vi "CRYPEAQ Makeing HarmonicTrack FlFcFu.vi"(10 "Harmonic Infor":T1={"Cycles"=[200.0, 190.0, 180.0, 170.0, 160.0, 150.0, 140.0, 132.0, 125.0, 118.0, 112.0, 106.0, 100.0, 95.0, 90.0, 85.0, 80.0, 75.0, 71.0, 67.0, 63.0, 60.0, 56.0, 53.0, 50.0, 48.0, 45.0, 43.0, 40.0, 38.0, 36.0, 34.0, 32.0, 30.0, 28.0, 27.0, 25.0, 24.0, 23.0, 22.0, 20.0, 19.0, 18.0, 17.0, 16.0, 15.0, 14.0, 14.0, 13.0, 12.0, 12.0, 11.0, 10.0, 10.0, 9.0, 9.0, 8.0, 8.0, 8.0, 7.0, 7.0, 6.0, 6.0, 6.0, 6.0, 6.0, 6.0, 6.0, 6.0, 6.0, 6.0, 6.0, 6.0, 6.0, 8.0, 8.0, 8.0, 8.0, 8.0, 8.0, 8.0, 8.0], "Frequency"=[20000.0, 19000.0, 18000.0, 17000.0, 16000.0, 15000.0, 14000.0, 13199.999809265137, 12500.0, 11800.000190734863, 11199.999809265137, 10600.000381469727, 10000.0, 9500.0, 9000.0, 8500.0, 8000.0, 7500.0, 7099.999904632568, 6699.999809265137, 6300.000190734863, 6000.0, 5599.999904632568, 5300.000190734863, 5000.0, 4750.0, 4500.0, 4250.0, 4000.0, 3750.0, 3549.999952316284, 3349.9999046325684, 3150.0000953674316, 3000.0, 2799.999952316284, 2650.0000953674316, 2500.0, 2359.999895095825, 2240.000009536743, 2119.999885559082, 2000.0, 1900.0, 1800.0, 1700.0, 1600.0, 1500.0, 1400.0, 1319.9999809265137, 1250.0, 1180.0000190734863, 1119.9999809265137, 1060.0000381469727, 1000.0, 950.0, 900.0, 850.0, 800.0, 750.0, 709.9999904632568, 669.9999809265137, 630.0000190734863, 600.0, 559.9999904632568, 530.0000190734863, 500.0, 475.0, 450.0, 425.0, 400.0, 375.0, 354.9999952316284, 334.99999046325684, 315.00000953674316, 300.0, 250.0, 200.0, 160.0, 125.0, 100.0, 80.0, 63.00000190734863, 50.0], "Amplitude"=[0.5, 0.5, 0.5, 0.5, 0.5, 0.5, 0.5, 0.5, 0.5, 0.5, 0.5, 0.5, 0.5, 0.5, 0.5, 0.5, 0.5, 0.5, 0.5, 0.5, 0.5, 0.5, 0.5, 0.5, 0.5, 0.5, 0.5, 0.5, 0.5, 0.5, 0.5, 0.5, 0.5, 0.5, 0.5, 0.5, 0.5, 0.5, 0.5, 0.5, 0.5, 0.5, 0.5, 0.5, 0.5, 0.5, 0.5, 0.5, 0.5, 0.5, 0.5, 0.5, 0.5, 0.5, 0.5, 0.5, 0.5, 0.5, 0.5, 0.5, 0.5, 0.5, 0.5, 0.5, 0.5, 0.5, 0.5, 0.5, 0.5, 0.5, 0.5, 0.5, 0.5, 0.5, 0.5, 0.5, 0.5, 0.5, 0.5, 0.5, 0.5, 0.5], "samples"=[441, 441, 441, 441, 441, 441, 441, 441, 441, 441, 441, 441, 441, 441, 441, 441, 441, 441, 441, 441, 441, 441, 441, 441, 441, 446, 441, 446, 441, 447, 447, 447, 448, 441, 441, 450, 441, 448, 453, 458, 441, 441, 441, 441, 441, 441, 441, 467, 459, 448, 473, 458, 441, 464, 441, 467, 441, 470, 497, 461, 490, 441, 472, 499, 530, 557, 588, 622, 662, 705, 746, 790, 840, 882, 1411, 1764, 2205, 2823, 3528, 4410, 5600, 7055], "Fs"=44100.0, "window"=7, "discard cycles"=1.0} {"discard cycles" min=1.0}) -> (0 "Max Frequency":dbl, 1 "Fu":dbl[](array[numeric])=[22.454773997922736, 22.97758714371529, 23.51258021383542, 24.060036879710538, 24.6202474215474, 25.193508881725744, 25.780125222574476, 26.380407487261397, 26.99467396487717, 27.62325035931701, 28.26646996176788, 28.92467382730014, 29.598210956047147, 30.287438477900952, 30.992721842290486, 31.714435011380765, 32.452960658853264, 33.208690372401655, 33.98202486161858, 34.773374170387285, 35.58315789437015, 36.41180540330013, 37.259756068478765, 38.127459496456304, 39.01537576663182, 39.923975675444694, 40.85374098616558, 41.80516468428786, 42.77875123862532, 43.77501686920085, 44.79448982064225, 45.83771064227755, 46.90523247502523, 47.99762134429284, 49.115456460467634, 50.2593305257138, 51.42985004836605, 52.62763566442533, 53.85332246665549, 55.10756034167334, 56.391014313751576, 57.70436489820836, 59.04830846170678, 60.423557591748676, 61.830841474273164, 63.27090628064966, 64.74451556287737, 66.25245065877897, 67.79551110590032, 69.37451506590403, 70.9902997579681, 72.64372190278358, 74.33565817714842, 76.0670056781684, 77.83868239945207, 79.65162771770717, 81.50680289034209, 83.40519156605784, 85.34780030545036, 87.33565911540498, 89.36982199479563, 91.45136749348208, 93.58139928410841, 95.76104674749965, 97.99146557116102, 100.27383836227469, 102.60937527440015, 104.99931464986868, 107.44492367538494, 109.94749905452376, 112.5083676952281, 115.12888741310817, 117.8104476515396, 120.55447021846123, 123.36241003987485, 126.23575593174236, 129.1760313889854, 132.18479539348297, 135.26364324037172, 138.4142073845422, 141.63815830533997, 144.93720539296265, 148.31309785436, 151.76762564113122, 155.30262039792564, 158.91995643433984, 162.62155171801825, 166.4093688923503, 170.2854163162711, 174.251749129759, 178.31047034303583, 182.46373195196514, 186.71373607895154, 191.06273614043988, 195.51303804181413, 200.06700139989707, 204.72704079434857, 209.49562704746577, 214.37528853468135, 219.3686125246637, 224.47824655161554, 229.70689981887307, 235.057344635006, 240.53241788431615, 246.135022530637, 251.86812915653312, 257.73477753839944, 263.73807825806085, 269.881214352571, 276.1674430011124, 282.6000972524956, 289.18258779245804, 295.91840475156465, 302.81111955630627, 309.8643868222997, 317.081946292187, 324.4676248185348, 332.0253383927343, 339.75909422140023, 347.67299285107083, 355.7712303422073, 364.0581004944929, 372.5379971226333, 381.2154163868554, 390.0949591762076, 399.1813335484587, 408.47935722609816, 417.99396015083505, 427.7301870974983, 437.6932003488361, 447.8882824328153, 458.3208389232213, 468.99640130595765, 479.92062991154586, 491.09931691702474, 502.5383894162503, 514.2439125630955, 526.2220927869496, 538.4792810835186, 551.0219763824239, 563.8568289927026, 576.9906441289077, 590.4303855198066, 604.1831790999819, 618.2563167885307, 632.6572603549645, 647.3936453762086, 662.4732852843022, 677.9041755094981, 693.6944977199626, 709.8526241591744, 726.387122085026, 743.3067583130218, 760.6205038636788, 778.3375387195264, 796.4672566926057, 815.0192704046698, 834.0034163843833, 853.429760282622, 873.3086022095733, 893.6504821954353, 914.4661857797167, 935.7667497292374, 957.5634678900275, 979.8678971760271, 1002.6918636957867, 1026.0474690237668, 1049.9470966162373, 1074.4034183769784, 1099.429401376779, 1125.0383147279376, 1151.2437366204622, 1178.059561520769, 1205.5000075390842, 1233.5796239681415, 1262.3132989970838, 1291.716267605563, 1321.8041196417378, 1352.592808087576, 1384.0986575181541, 1416.3383727566554, 1449.329047731571, 1483.0881745401007, 1517.6336527227509, 1552.983798754135, 1589.1573557540758, 1626.173503426001, 1664.0518682259462, 1702.8125337688543, 1742.4760514771751, 1783.0634514774647, 1824.596253750986, 1867.0964795436084, 1910.5866630422083, 1955.0898633219676, 2000.629676573275, 2047.2302486121253, 2094.916287683119, 2143.7130775595638, 2193.6464909496717, 2244.7430032145617, 2297.0297064054575, 2350.534323628789, 2405.2852237450925, 2461.3114364103076, 2518.642667468382, 2577.309314700866, 2637.342483944817, 2698.774005585298, 2761.636451432274, 2825.9631519907193, 2891.788214132709, 2959.1465391814268, 3028.073841416658, 3098.6066670100945, 3170.7824134035327, 3244.6393491370727, 3320.21663413942, 3397.554340491384, 3476.69347367248, 3557.675994302525, 3640.544840389543, 3725.3439500966592, 3812.118285038006, 3900.9138541182183, 3991.777737927235, 4084.7581137026004, 4179.904280874161, 4277.266687202766, 4376.896955528673, 4478.84791114254, 4583.173609794229, 4689.9293663536055, 4799.17178413954, 4910.958784931605, 5025.349639680679, 5142.40499993584, 5262.186930001873, 5384.7589398471655, 5510.186018777306, 5638.534669893191, 5769.872945352114, 5904.270482449578, 6041.798540542085, 6182.530038829943, 6326.539595019659, 6473.903564887547, 6624.700082764322, 6779.009102963305, 6936.912442172715, 7098.493822836377, 7263.838917544618, 7433.0353944582685, 7606.172963792461, 7783.34342538143, 7964.640717352117, 8150.16096593186, 8340.002536415303, 8534.266085318994, 8733.05461375138, 8936.473522024511, 9144.630665539245, 9357.636411971636, 9575.60369979094, 9798.648098141424, 18000.0] format="%#.6g", 2 "Fc":dbl[](array[numeric]), 3 "Fl":dbl[](array[numeric])=[20.0, 22.454773997922736, 22.97758714371529, 23.51258021383542, 24.060036879710538, 24.6202474215474, 25.193508881725744, 25.780125222574476, 26.380407487261397, 26.99467396487717, 27.62325035931701, 28.26646996176788, 28.92467382730014, 29.598210956047147, 30.287438477900952, 30.992721842290486, 31.714435011380765, 32.452960658853264, 33.208690372401655, 33.98202486161858, 34.773374170387285, 35.58315789437015, 36.41180540330013, 37.259756068478765, 38.127459496456304, 39.01537576663182, 39.923975675444694, 40.85374098616558, 41.80516468428786, 42.77875123862532, 43.77501686920085, 44.79448982064225, 45.83771064227755, 46.90523247502523, 47.99762134429284, 49.115456460467634, 50.2593305257138, 51.42985004836605, 52.62763566442533, 53.85332246665549, 55.10756034167334, 56.391014313751576, 57.70436489820836, 59.04830846170678, 60.423557591748676, 61.830841474273164, 63.27090628064966, 64.74451556287737, 66.25245065877897, 67.79551110590032, 69.37451506590403, 70.9902997579681, 72.64372190278358, 74.33565817714842, 76.0670056781684, 77.83868239945207, 79.65162771770717, 81.50680289034209, 83.40519156605784, 85.34780030545036, 87.33565911540498, 89.36982199479563, 91.45136749348208, 93.58139928410841, 95.76104674749965, 97.99146557116102, 100.27383836227469, 102.60937527440015, 104.99931464986868, 107.44492367538494, 109.94749905452376, 112.5083676952281, 115.12888741310817, 117.8104476515396, 120.55447021846123, 123.36241003987485, 126.23575593174236, 129.1760313889854, 132.18479539348297, 135.26364324037172, 138.4142073845422, 141.63815830533997, 144.93720539296265, 148.31309785436, 151.76762564113122, 155.30262039792564, 158.91995643433984, 162.62155171801825, 166.4093688923503, 170.2854163162711, 174.251749129759, 178.31047034303583, 182.46373195196514, 186.71373607895154, 191.06273614043988, 195.51303804181413, 200.06700139989707, 204.72704079434857, 209.49562704746577, 214.37528853468135, 219.3686125246637, 224.47824655161554, 229.70689981887307, 235.057344635006, 240.53241788431615, 246.135022530637, 251.86812915653312, 257.73477753839944, 263.73807825806085, 269.881214352571, 276.1674430011124, 282.6000972524956, 289.18258779245804, 295.91840475156465, 302.81111955630627, 309.8643868222997, 317.081946292187, 324.4676248185348, 332.0253383927343, 339.75909422140023, 347.67299285107083, 355.7712303422073, 364.0581004944929, 372.5379971226333, 381.2154163868554, 390.0949591762076, 399.1813335484587, 408.47935722609816, 417.99396015083505, 427.7301870974983, 437.6932003488361, 447.8882824328153, 458.3208389232213, 468.99640130595765, 479.92062991154586, 491.09931691702474, 502.5383894162503, 514.2439125630955, 526.2220927869496, 538.4792810835186, 551.0219763824239, 563.8568289927026, 576.9906441289077, 590.4303855198066, 604.1831790999819, 618.2563167885307, 632.6572603549645, 647.3936453762086, 662.4732852843022, 677.9041755094981, 693.6944977199626, 709.8526241591744, 726.387122085026, 743.3067583130218, 760.6205038636788, 778.3375387195264, 796.4672566926057, 815.0192704046698, 834.0034163843833, 853.429760282622, 873.3086022095733, 893.6504821954353, 914.4661857797167, 935.7667497292374, 957.5634678900275, 979.8678971760271, 1002.6918636957867, 1026.0474690237668, 1049.9470966162373, 1074.4034183769784, 1099.429401376779, 1125.0383147279376, 1151.2437366204622, 1178.059561520769, 1205.5000075390842, 1233.5796239681415, 1262.3132989970838, 1291.716267605563, 1321.8041196417378, 1352.592808087576, 1384.0986575181541, 1416.3383727566554, 1449.329047731571, 1483.0881745401007, 1517.6336527227509, 1552.983798754135, 1589.1573557540758, 1626.173503426001, 1664.0518682259462, 1702.8125337688543, 1742.4760514771751, 1783.0634514774647, 1824.596253750986, 1867.0964795436084, 1910.5866630422083, 1955.0898633219676, 2000.629676573275, 2047.2302486121253, 2094.916287683119, 2143.7130775595638, 2193.6464909496717, 2244.7430032145617, 2297.0297064054575, 2350.534323628789, 2405.2852237450925, 2461.3114364103076, 2518.642667468382, 2577.309314700866, 2637.342483944817, 2698.774005585298, 2761.636451432274, 2825.9631519907193, 2891.788214132709, 2959.1465391814268, 3028.073841416658, 3098.6066670100945, 3170.7824134035327, 3244.6393491370727, 3320.21663413942, 3397.554340491384, 3476.69347367248, 3557.675994302525, 3640.544840389543, 3725.3439500966592, 3812.118285038006, 3900.9138541182183, 3991.777737927235, 4084.7581137026004, 4179.904280874161, 4277.266687202766, 4376.896955528673, 4478.84791114254, 4583.173609794229, 4689.9293663536055, 4799.17178413954, 4910.958784931605, 5025.349639680679, 5142.40499993584, 5262.186930001873, 5384.7589398471655, 5510.186018777306, 5638.534669893191, 5769.872945352114, 5904.270482449578, 6041.798540542085, 6182.530038829943, 6326.539595019659, 6473.903564887547, 6624.700082764322, 6779.009102963305, 6936.912442172715, 7098.493822836377, 7263.838917544618, 7433.0353944582685, 7606.172963792461, 7783.34342538143, 7964.640717352117, 8150.16096593186, 8340.002536415303, 8534.266085318994, 8733.05461375138, 8936.473522024511, 9144.630665539245, 9357.636411971636, 9575.60369979094, 9798.648098141424] format="%#.6g")   [LabVIEW 2013]
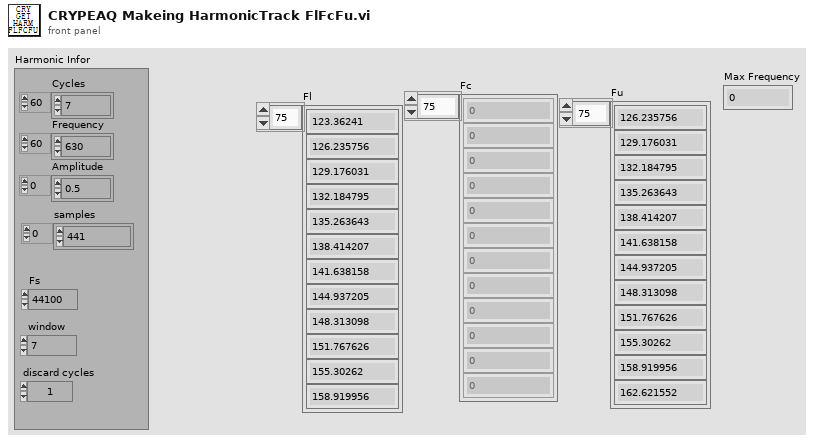
[diagram p1: front panel]
types:
  T1 = cluster{"Cycles":dbl[], "Frequency":dbl[], "Amplitude":dbl[], "samples":i32[], "Fs":dbl, "window":u16, "discard cycles":dbl}
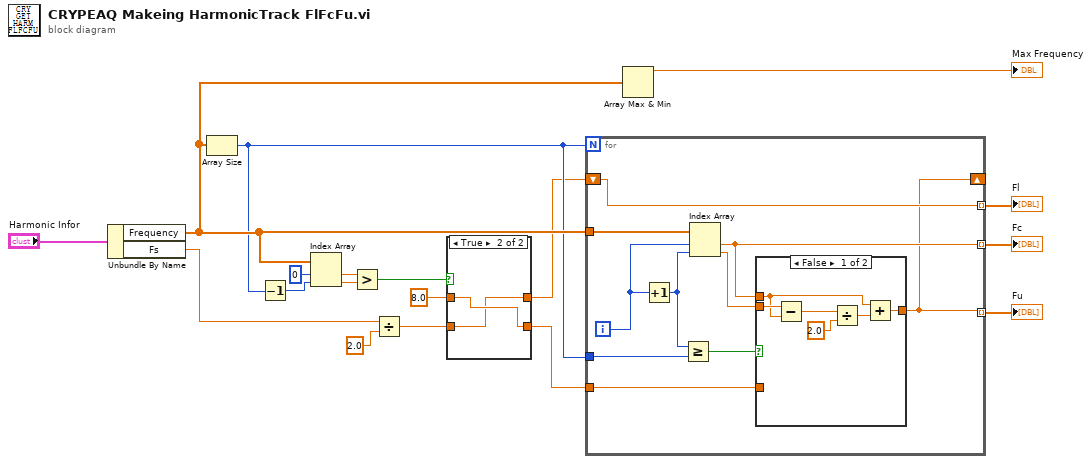
[diagram p0: block diagram]
diagram:
  n1 = Unbundle By Name("Harmonic Infor") -> ("Frequency"=w11:dbl[], "Fs"=w17:dbl)
  n2 = Array Size(array=w11) -> (size(s)=w9:i32)
  n3 = Decrement(x=w9) -> (x-1=w8:i32)
  n4 = Index Array(array=w11, index #1=0 ("index"), index #2=w8) -> (element #1=w7:dbl, element #2=w6:dbl)
  n5 = Greater?(x=w7, y=w6) -> (0:w5:bool)
  n6 = Divide(x=w17, y=2.0) -> (x/y=w4:dbl)
  n7 = case shown="True" w5 {
    tunnel: w4 -> [w19 w21]
    tunnel: 8.0 ("y") -> [w20 w22]
    tunnel: [w19 w22] -> w2
    tunnel: [w20 w21] -> w1
    frame False {
    }
    frame True {
    }
  }
  n8 = for {
    N: w9 -> [_]
    tunnel: w11 -> [w31]
    shift-right: [w27] -> _
    shift-left: w1 -> [w32]
    tunnel: [w32] -> w15 mode=indexing
    tunnel: [w28] -> w14 mode=indexing
    tunnel: [w27] -> w13 mode=indexing
    tunnel: w9 -> [w26]
    tunnel: w2 -> [w23]
    i -> [w30]
    n9 = Increment(x=w30) -> (x+1=w25:i32)
    n10 = Greater Or Equal?(x=w25, y=w26) -> (x >= y?=w24:bool)
    n11 = Index Array(array=w31, index #1=w30, index #2=w25) -> (element #1=w28:dbl, element #2=w29:dbl)
    n12 = case shown="False" w24 {
      tunnel: w29 -> [w38 _]
      tunnel: w28 -> [w35 _]
      tunnel: [w33 w39] -> w27
      tunnel: w23 -> [_ w39]
      frame False {
        n13 = Subtract(x=w38, y=w35) -> (x-y=w37:dbl)
        n14 = Divide(x=w37, y=2.0) -> (x/y=w34:dbl)
        n15 = Add(x=w35, y=w34) -> (x+y=w33:dbl)
      }
      frame True {
      }
    }
  }
  "Fu" <- w13
  "Fl" <- w15
  "Fc" <- w14
  n16 = Array Max & Min(array=w11) -> (max value=→"Max Frequency":dbl)  [unwired: 3 out]
